vi "Signal_acquisition_v5.vi"() -> ()   [LabVIEW 2015]
uses:
  <vilib>/measure/madcrms.llb/Basic Averaged DC-RMS for 1 Chan.vi
  <vilib>/measure/matone.llb/Extract Single Tone Information 1 Chan.vi
  <vilib>/express/express arith-compare/Formula/XNode/ExpressFormulaBlockNode.xnode
  <vilib>/measure/NI_MAPro.lvlib
panel:
  in  "timeout ms":i32=2000
  in  "timeout ms\n (2000)":i32=2000
  in  "timeout ms\n (2000) 2":i32=2000
  in  "Delay\n (# Samples)":i32 max=16348
  in  "Trigger Level \n(0 mV)":i32
  out "DC value 2":dbl format="%0.2p"
  out "detected \nfrequency 2":dbl format="%.2p"
  out "Ieration\nnumber":i32
  out "millisecond \ntimer value":u32
  out "millisecond \nbegin timer":u32
  out "millisecond \nfinal timer":u32
  in  "Tab Control":T1(tab)
  out "Voltage Gain / Frequency":cluster{i32, dbl}[](graph)
  out "Cutoff Freqs (Hz)":i32[](array[numeric])
  in  "MEASURE AMPLITUD":bool
  out "Acquisition\ntime complete":u32
  out "MEASURED \namplitud":dbl format="%.2p"
  out "RESULT \nin amplittude":dbl
  out "FRECUENCY \nEND":i32
  out "detected \nphase (deg)":dbl format="%.2p"
  out "detected \nfrequency":dbl format="%.2p"
  in  "Filename":path=path "test.xlsx"
  in  "Trigger Mode":string(combo)="CH1_NE"
  in  "input":u16=1
  in  "Pause \nfor buffer (ms)":u32=100
  out "error out":errorcluster
  in  "VOLTS":dbl=0.1
  in  "FREQ END":i32=70000
  in  "FREQ START":i32=10000
  in  "number \nof intervals":i32=60
  in  "IP address":string="192.168.0.10"
  in  "Decimation":u16(ring)=8 items=["65536"=65535, "8192"=8192, "1024"=1024, "64"=64, "8"=8, "1"=1]
  in  "error in":errorcluster
  out "REAL TIME MEASUREMENT":dbl[](graph)
  in  "FREQ START 5":i32
  in  "number of intervals  3":i32
  in  "number of intervals  2":i32
  # "FREQUENCY SWEEP"
  # "FREQUENCY SWEEP"
  # "Settings parameters"
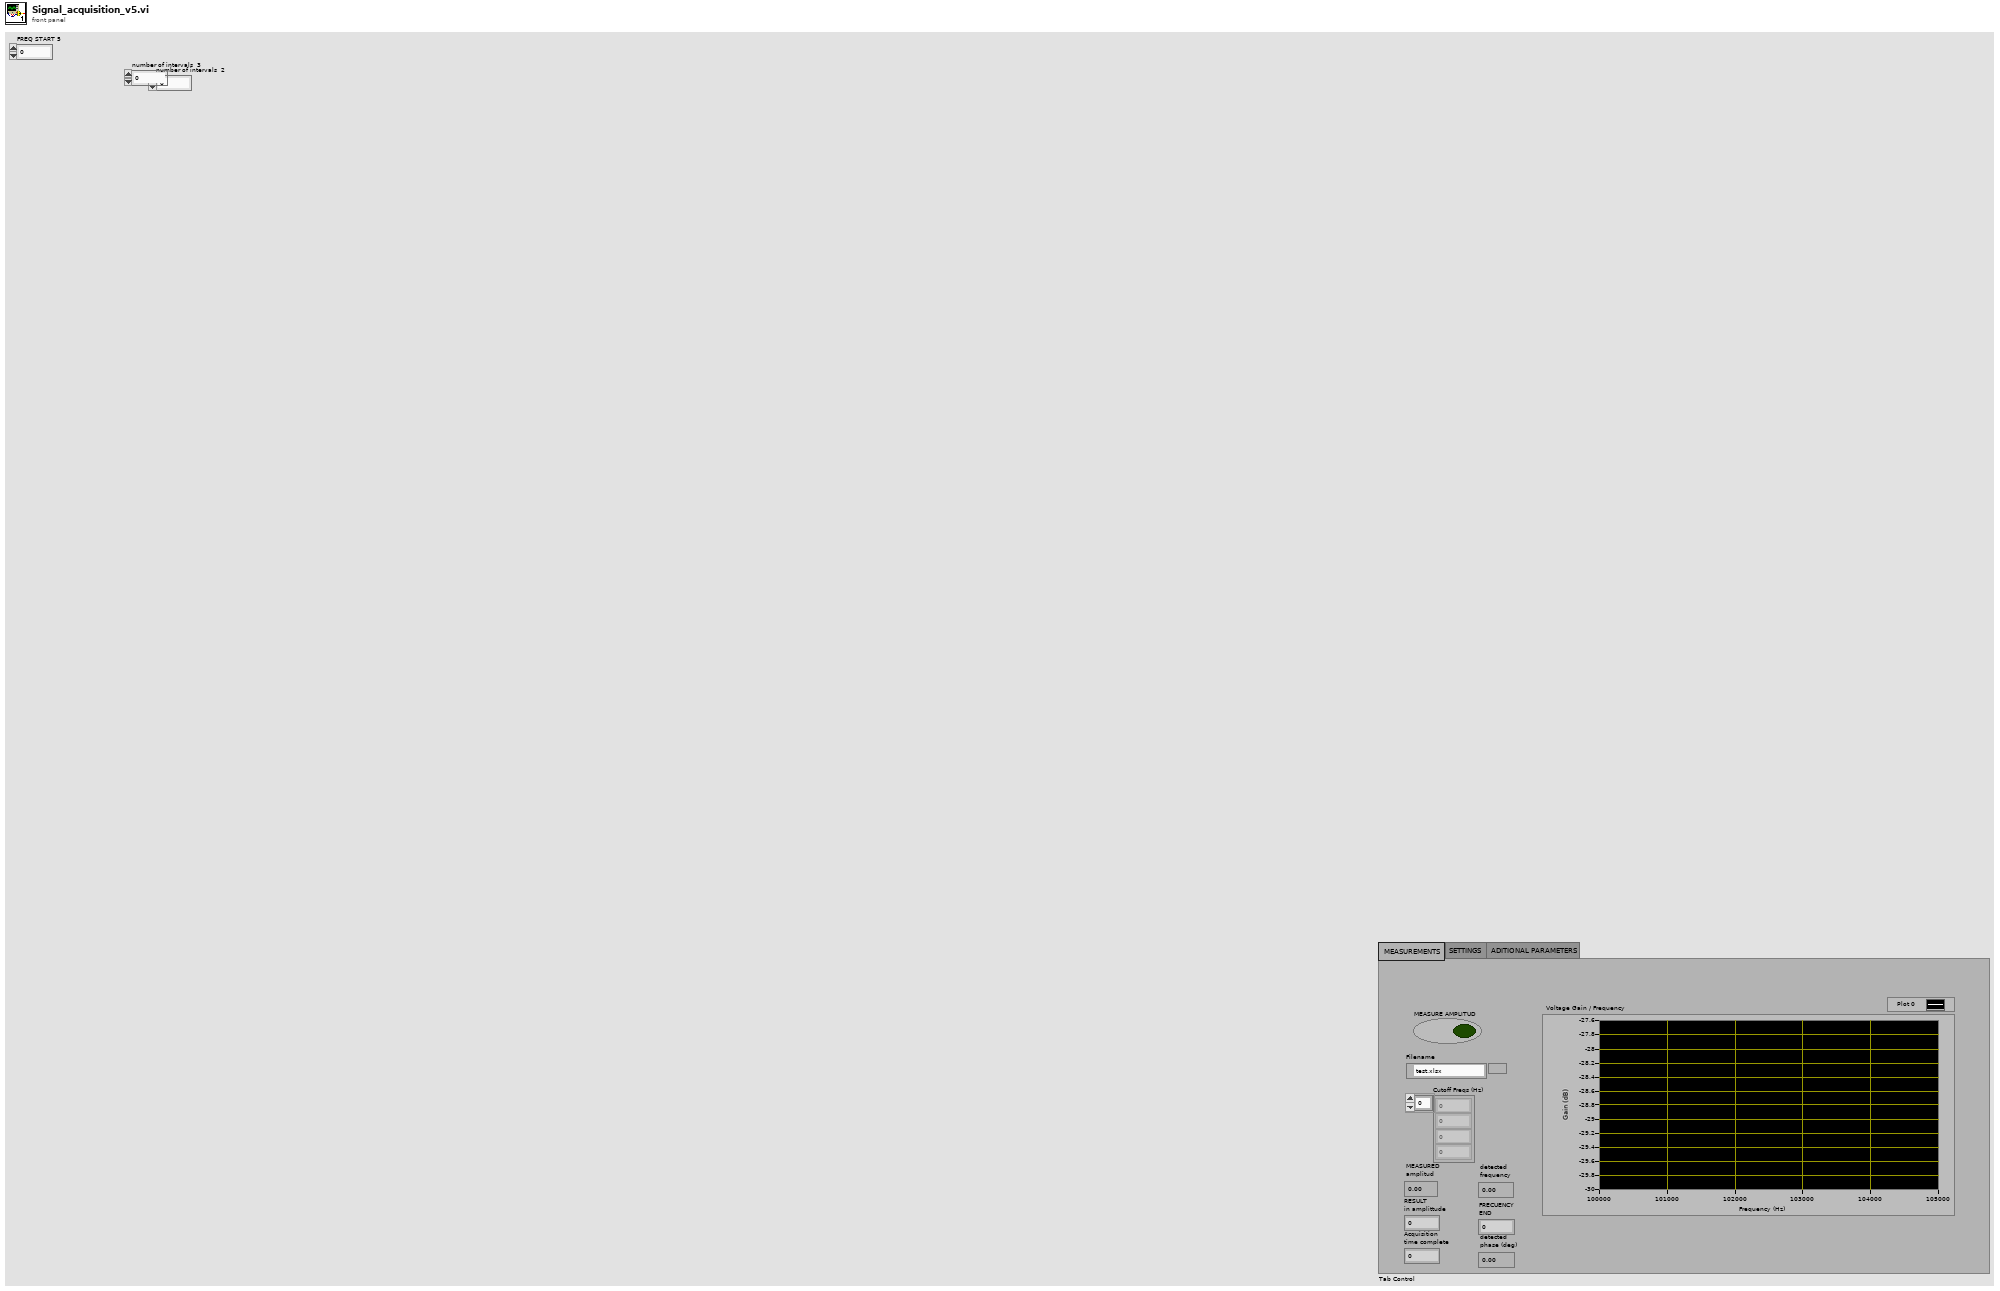
[diagram p1: front panel]
types:
  T1 = enum32{"MEASUREMENTS ", "SETTINGS", "ADITIONAL PARAMETERS"}
  T2 = enum16{"Standard", "Buffered", "CRLF", "Immediate"}
  T3 = enum32{"none", "input signal", "detected signal", "residual signal"}
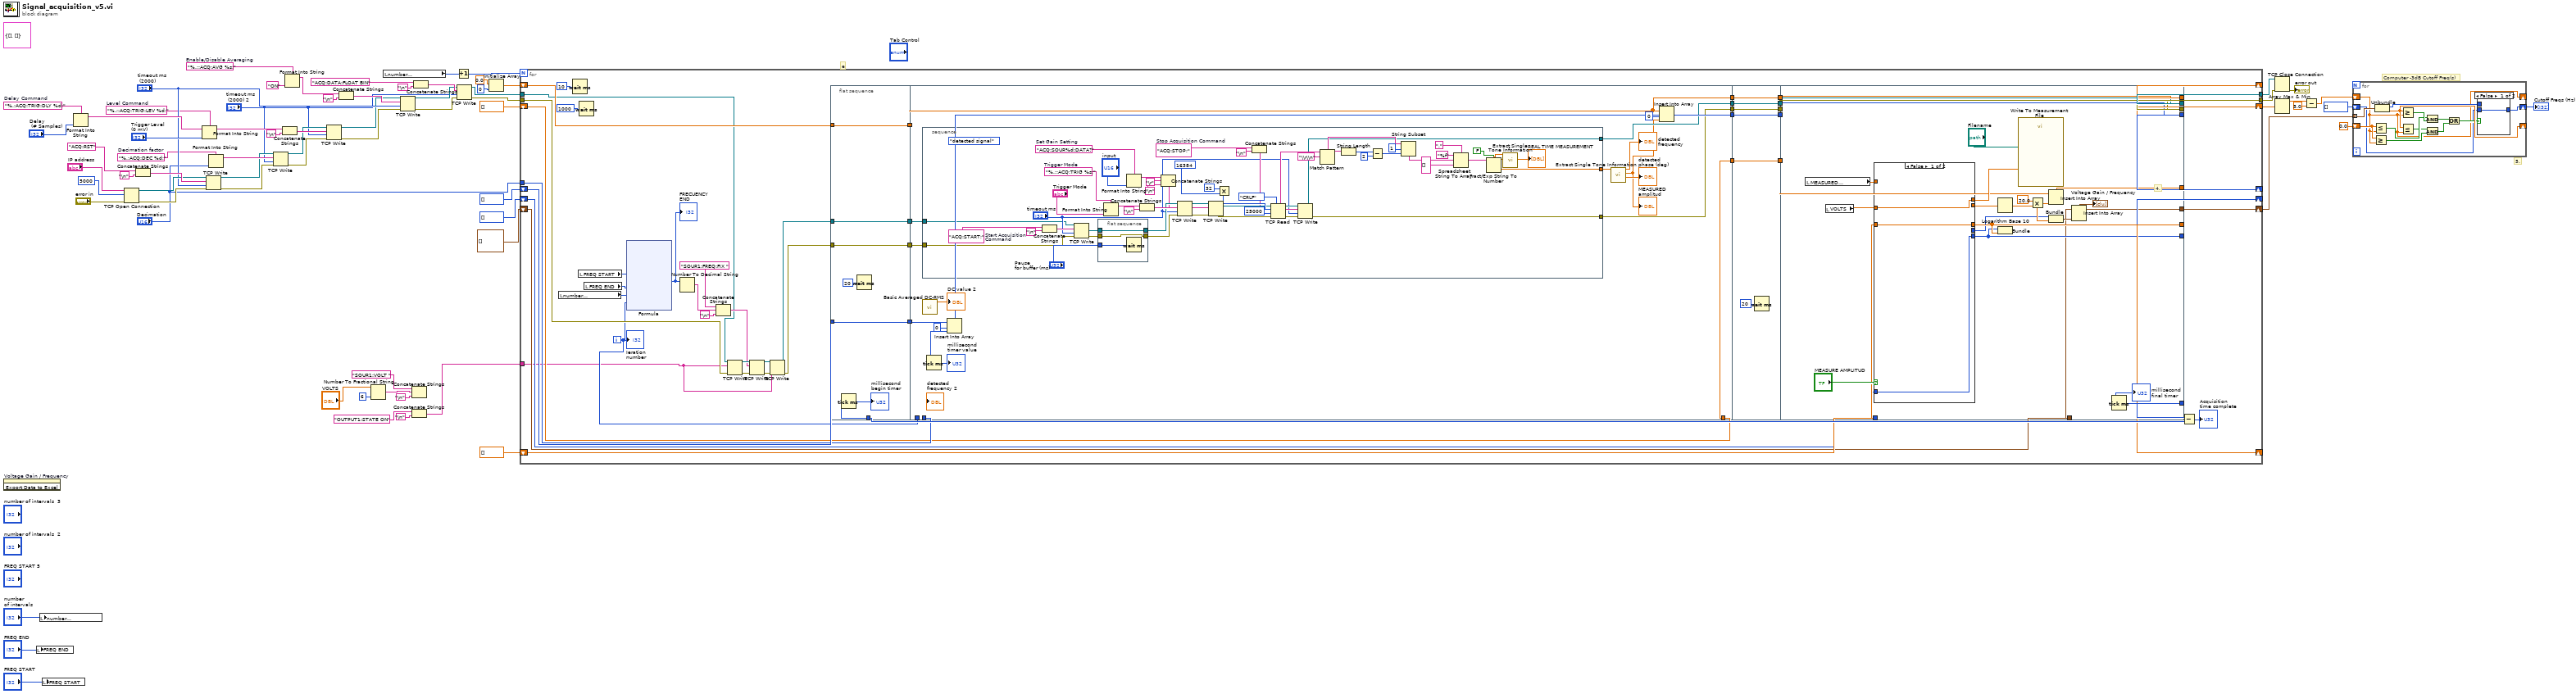
[diagram p0: block diagram]
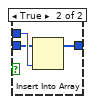
[diagram p2: hidden frame]
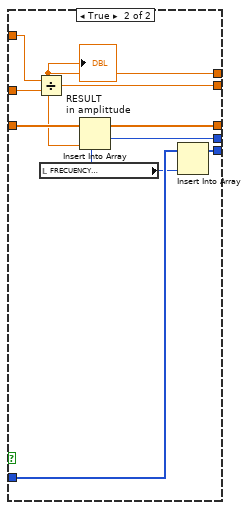
[diagram p3: hidden frame]
diagram:
  (unwired) cluster{dbl[], dbl[]} {[], []} ("FRECUENCY SWEEP")
  w37 = "%.;:ACQ:AVG %s;"  # Enable/Disable Averaging
  w45 = "%.;ACQ:DEC %d;"  # Decimation factor
  w46 = "%.;ACQ:TRIG:DLY %d;"  # Delay Command
  w47 = "%.;:ACQ:TRIG:LEV %d;"  # Level Command
  # "5."
  # "Computer -3dB Cutoff Freq(s)"
  # "e"
  n1 = invoke on="Voltage Gain / Frequency" class="XYGraph (strict)" method="Export Data to Excel"() -> ()  [unwired: 3 in, 3 out]
  n2 = local write "FREQ END"("FREQ END") -> ()
  n3 = local write "number \nof intervals"("number \nof intervals") -> ()
  n4 = local write "FREQ START"("FREQ START") -> ()
  n5 = Format Into String(format string=w46, "Delay\n (# Samples)") -> (resulting string=w65:string)  [unwired: 2 in, 1 out]
  n6 = TCP Open Connection(address="IP address", remote port or service name=u16 5000, error in (no error)="error in") -> (connection ID=w59:refnum<k5>, error out=w58:errorcluster)  [unwired: 2 in]
  n7 = Concatenate Strings("ACQ:RST" ("SCPI Message"), "\n") -> (w61:string)
  n8 = Format Into String(format string=w47, initial string=w65, "Trigger Level \n(0 mV)") -> (resulting string=w62:string)  [unwired: 1 in, 1 out]
  n9 = TCP Write(connection ID=w59, data in=w61, error in (no error)=w58, 9:"timeout ms\n (2000)") -> (connection ID out=w43:refnum<k5>, error out=w42:errorcluster)  [unwired: 1 out]
  n10 = Format Into String(format string=w45, "Decimation") -> (resulting string=w44:string)  [unwired: 2 in, 1 out]
  n11 = TCP Write(connection ID=w43, data in=w44, error in (no error)=w42, 9:"timeout ms\n (2000) 2") -> (connection ID out=w41:refnum<k5>, error out=w40:errorcluster)  [unwired: 1 out]
  n12 = Concatenate Strings(w62, "\n") -> (w56:string)
  n13 = Format Into String(format string=w37, "ON") -> (resulting string=w68:string)  [unwired: 2 in, 1 out]
  n14 = TCP Write(connection ID=w41, data in=w56, error in (no error)=w40, 9:"timeout ms\n (2000) 2") -> (connection ID out=w39:refnum<k5>, error out=w38:errorcluster)  [unwired: 1 out]
  n15 = Concatenate Strings(w68, "\n") -> (w57:string)
  n16 = Number To Fractional String(number="VOLTS", precision (6)=i16 6) -> (F-format string=w7:string)  [unwired: 2 in]
  n17 = local read "number \nof intervals"() -> (w23:i32)
  n18 = TCP Write(connection ID=w39, data in=w57, error in (no error)=w38, 9:"timeout ms\n (2000)") -> (connection ID out=w35:refnum<k5>, error out=w34:errorcluster)  [unwired: 1 out]
  n19 = Concatenate Strings("SOUR1:VOLT " ("SCPI Message"), w7, "\n") -> ()  [unwired: 1 out]
  n20 = Concatenate Strings("OUTPUT1:STATE ON" ("SCPI Message"), "\n") -> (w1:string)
  n21 = Concatenate Strings("ACQ:DATA:FLOAT BIN" ("SCPI Message"), "\n") -> (w53:string)
  n22 = Increment(x=w23) -> (x+1=w22:i32)
  n23 = TCP Write(connection ID=w35, data in=w53, error in (no error)=w34, 9:"timeout ms\n (2000) 2") -> (connection ID out=w32:refnum<k5>, error out=w31:errorcluster)  [unwired: 1 out]
  n24 = Initialize Array(0.0 ("element"), 0 ("dimension size")) -> (w26:dbl[])
  n25 = for {
    N: w22 -> [_]
    tunnel: w32 -> [w103]
    tunnel: [w121] -> w52
    tunnel: [w120] -> w51
    tunnel: w31 -> [w100]
    shift-right: [w123] -> _
    shift-left: u32[] [] -> [w122]
    tunnel: "Decimation" -> [w113]
    shift-right: [w111] -> _
    shift-left: w26 -> [w109]
    shift-right: [w96] -> _
    shift-left: dbl[] [] -> [w97]
    shift-right: [w92] -> _
    shift-left: i32[] [] -> [w91]
    shift-right: [w87] -> w11
    shift-left: dbl[] [] -> [w86]
    shift-right: [w85] -> w10
    shift-left: cluster{"FRECUENCY END":i32, dbl}[] [] -> [w84]
    tunnel: w1 -> [w72]
    i -> [w73]
    n26 = local read "number \nof intervals"() -> (w93:i32)
    n27 = Wait (ms)(milliseconds to wait=u32 10) -> ()  [unwired: 1 out]
    n28 = local read "FREQ START"() -> (w94:i32)
    n29 = Wait (ms)(milliseconds to wait=u32 1000) -> ()  [unwired: 1 out]
    n30 = local read "FREQ END"() -> (w95:i32)
    n31 = xnode "Formula"("Fin"=w94, "Fend"=w95, "Ninter"=w93, "i"=w73) -> ("Result"=w88:i32)  [unwired: 1 in, 1 out]
    "FRECUENCY \nEND" <- w88
    n32 = Number To Decimal String(number=w88) -> (decimal integer string=w98:string)  [unwired: 1 in]
    n33 = Concatenate Strings("SOUR1:FREQ:FIX " ("SCPI Message"), w98, "\n") -> (w104:string)
    n34 = TCP Write(connection ID=w103, data in=w72, error in (no error)=w100) -> (connection ID out=w107:refnum<k5>, error out=w106:errorcluster)  [unwired: 1 in, 1 out]
    n35 = TCP Write(connection ID=w107, data in=w104, error in (no error)=w106) -> (connection ID out=w90:refnum<k5>, error out=w89:errorcluster)  [unwired: 1 in, 1 out]
    n36 = TCP Write(connection ID=w90, data in=w72, error in (no error)=w89) -> (connection ID out=w102:refnum<k5>, error out=w101:errorcluster)  [unwired: 1 in, 1 out]
    n37 = flat-sequence {
      tunnel: w122 -> [w141]
      tunnel: w101 -> [w142]
      tunnel: w102 -> [w143]
      tunnel: [w143] -> w119
      tunnel: [w142] -> w118
      tunnel: [w141] -> w117
      tunnel: [w140] -> w115
      tunnel: [w139] -> w110
      tunnel: w109 -> [w139]
      tunnel: [w155] -> w83
      tunnel: [w153] -> w81
      tunnel: [w152] -> w79
      tunnel: w119 -> [w159]
      tunnel: w118 -> [w158]
      tunnel: w117 -> [w154]
      tunnel: w113 -> [_]
      tunnel: [w148] -> w77
      tunnel: w73 -> [_]
      tunnel: w110 -> [w148]
      tunnel: w86 -> [w144]
      tunnel: [w144] -> w75
      tunnel: w83 -> [w220]
      tunnel: [w220] -> w82
      tunnel: w81 -> [w219]
      tunnel: [w219] -> w80
      tunnel: w79 -> [w218]
      tunnel: [w218] -> w78
      tunnel: w77 -> [w217]
      tunnel: [w217] -> w76
      tunnel: w75 -> [w216]
      tunnel: [w216] -> w74
      tunnel: [w242] -> w120
      tunnel: [w243] -> w121
      tunnel: [w244] -> w123
      tunnel: w82 -> [w244]
      tunnel: w80 -> [w243]
      tunnel: w78 -> [w242]
      tunnel: [w241] -> w116
      tunnel: w76 -> [w240]
      tunnel: [w240] -> w111
      tunnel: w97 -> [w236]
      tunnel: [w234] -> w96
      tunnel: [w233] -> w92
      tunnel: w91 -> [w235]
      tunnel: [w228] -> w87
      tunnel: w74 -> [w227]
      tunnel: [w225] -> w85
      tunnel: w84 -> [w224]
      frame #0 {
        n38 = Tick Count (ms)() -> (millisecond timer value=w140:u32)
        "millisecond \nbegin timer" <- w140
        n39 = Wait (ms)(milliseconds to wait=u32 20) -> ()  [unwired: 1 out]
      }
      frame #1 {
        n40 = stacked-sequence {
          tunnel: w159 -> [w161]
          tunnel: w158 -> [w164]
          tunnel: [w162] -> w153
          tunnel: [w163] -> w152
          tunnel: [w160] -> w146
          frame #0 {
            w171 = "ACQ:STOP;"  # Stop Acquisition Command
            (unwired) T3."detected signal" ("export mode")
            w181 = "ACQ:SOUR%d:DATA?"  # Set Gain Setting
            w208 = "%.;:ACQ:TRIG %s;"  # Trigger Mode
            w210 = "ACQ:START;"  # Start Acquisition Command
            n41 = Concatenate Strings(w210, "\n") -> (w211:string)
            n42 = TCP Write(connection ID=w161, data in=w211, error in (no error)=w164, 9:"timeout ms") -> (connection ID out=w185:refnum<k5>, error out=w184:errorcluster)  [unwired: 1 out]
            n43 = flat-sequence {
              tunnel: "Pause \nfor buffer (ms)" -> [w214]
              tunnel: [w213] -> w183
              tunnel: [w212] -> w182
              tunnel: w185 -> [w213]
              tunnel: w184 -> [w212]
              frame #0 {
                n44 = Wait (ms)(milliseconds to wait=w214) -> ()  [unwired: 1 out]
              }
            }
            n45 = Format Into String(format string=w208, "Trigger Mode") -> (resulting string=w205:string)  [unwired: 2 in, 1 out]
            n46 = Format Into String(format string=w181, "input") -> (resulting string=w179:string)  [unwired: 2 in, 1 out]
            n47 = Concatenate Strings(w205, "\n") -> (w206:string)
            n48 = Concatenate Strings(w179, "\r", "\n") -> (w178:string)
            n49 = TCP Write(connection ID=w183, data in=w206, error in (no error)=w182, 9:"timeout ms") -> (connection ID out=w176:refnum<k5>, error out=w175:errorcluster)  [unwired: 1 out]
            n50 = TCP Write(connection ID=w176, data in=w178, error in (no error)=w175) -> (connection ID out=w177:refnum<k5>, error out=w174:errorcluster)  [unwired: 1 in, 1 out]
            n51 = Multiply(x=32, y=16384 ("bytes to read")) -> (x*y=w186:i32)
            n52 = Concatenate Strings(w171, "\n") -> (w169:string)
            n53 = TCP Read(connection ID=w177, bytes to read=w186, error in (no error)=w174, 7:T2."CRLF" ("mode (standard)"), 9:25000 ("timeout ms (25000)")) -> (connection ID out=w172:refnum<k5>, data out=w187:string, error out=w168:errorcluster)
            n54 = TCP Write(connection ID=w172, data in=w169, error in (no error)=w168, 9:"timeout ms") -> (connection ID out=w162:refnum<k5>, error out=w163:errorcluster)  [unwired: 1 out]
            n55 = Match Pattern(string=w187, regular expression="\\r\\n") -> (before substring=w193:string)  [unwired: 1 in, 3 out]
            n56 = String Length(string=w193) -> (length=w196:i32)
            n57 = Subtract(x=w196, y=2) -> (x-y=w197:i32)
            n58 = String Subset(string=w193, offset (0)=1, length (rest)=w197) -> (substring=w194:string)
            n59 = Spreadsheet String To Array(delimiter (Tab)=",", format string="%f", spreadsheet string=w194, array type (2D Dbl)=string[] [] ("Array")) -> (array=w200:string[])
            n60 = Fract/Exp String To Number(use system decimal point (T)=FALSE, string=w200) -> (number=w160:dbl[])  [unwired: 3 out]
            "REAL TIME MEASUREMENT" <- w160
            n61 = call-poly <vilib>:"Extract Single Tone Information.vi"("time signal in"=w160) -> ()  [unwired: 5 in, 6 out]
          }
        }
        n62 = call-poly <vilib>:"Basic Averaged DC-RMS.vi"() -> ("DC value"=→"DC value 2":dbl)  [unwired: 8 in, 3 out]
        n63 = Tick Count (ms)() -> (millisecond timer value=w156:u32)
        "millisecond \ntimer value" <- w156
        n64 = Insert Into Array(array=w154, index=0, new element=w156) -> (w155:u32[])
        n65 = call-poly <vilib>:"Extract Single Tone Information.vi"("time signal in"=w146) -> ("detected phase (deg)"=→"detected \nphase (deg)":dbl, "detected amplitude"=w145:dbl, "detected frequency"=→"detected \nfrequency":dbl)  [unwired: 5 in, 3 out]
        "MEASURED \namplitud" <- w145
        n66 = Insert Into Array(array=w148, index=0, new element=w145) -> ()  [unwired: 1 out]
      }
      frame #2 {
        n67 = Wait (ms)(milliseconds to wait=u32 20) -> ()  [unwired: 1 out]
      }
      frame #3 {
        # "4."
        n68 = local read "MEASURED \namplitud"() -> (w239:dbl)
        n69 = local read "VOLTS"() -> (w222:dbl)
        n70 = case shown="False" "MEASURE AMPLITUD" {
          tunnel: w239 -> [_ w251]
          tunnel: [w245 w250] -> w237
          tunnel: w236 -> [w247 w255]
          tunnel: [w247 w254] -> w234
          tunnel: [w246 w253] -> w233
          tunnel: w235 -> [w246 w252]
          tunnel: [_ w250] -> w223
          tunnel: [_ w249] -> w226
          tunnel: w222 -> [w245 w248]
          frame False {
          }
          frame True {
            n71 = Divide(x=w251, y=w248) -> (x/y=w250:dbl)
            "RESULT \nin amplittude" <- w250
            n72 = local read "FRECUENCY \nEND"() -> (w249:i32)
            n73 = Insert Into Array(array=w255, new element=w250) -> (w254:dbl[])  [unwired: 1 in]
            n74 = Insert Into Array(array=w252, new element=w249) -> (w253:i32[])  [unwired: 1 in]
          }
        }
        n75 = Logarithm Base 10(1:w223) -> (0:w230:dbl)
        n76 = Bundle(w233, w234) -> ()  [unwired: 1 in, 1 out]
        n77 = call "Write To Measurement File"("Signals"=w237, "Filename"="Filename") -> ()  [unwired: 15 in, 3 out]
        n78 = Multiply(x=20.0, y=w230) -> (x*y=w229:dbl)
        n79 = Insert Into Array(array=w227, new element=w229) -> (w228:dbl[])  [unwired: 1 in]
        n80 = Bundle("FRECUENCY \nEND"=w226, w229) -> (w232:cluster{"FRECUENCY \nEND":i32, dbl})  [unwired: 1 in]
        n81 = Insert Into Array(array=w224, new element=w232) -> (w225:cluster{"FRECUENCY END":i32, dbl}[])  [unwired: 1 in]
        "Voltage Gain / Frequency" <- w225
        n82 = Tick Count (ms)() -> (millisecond timer value=w241:u32)
        "millisecond \nfinal timer" <- w241
      }
    }
    n83 = Subtract(x=w116, y=w115) -> (x-y=→"Acquisition\ntime complete":u32)
    "Ieration\nnumber" <- w73
  }
  n84 = TCP Close Connection(connection ID=w52, error in (no error)=w51) -> (error out=→"error out":errorcluster)  [unwired: 1 in, 1 out]
  n85 = Array Max & Min(array=w11) -> (max value=w12:dbl)  [unwired: 3 out]
  n86 = Subtract(x=w12, y=3.0) -> (x-y=w13:dbl)
  n87 = for {
    tunnel: w10 -> [w269] mode=indexing
    shift-right: [w263] -> _
    shift-left: 0.0 -> [w264]
    shift-right: [w257] -> w15
    shift-left: i32[] [] -> [w258]
    shift-right: [w256] -> _
    shift-left: w13 -> [w256]
    n88 = Less Or Equal?(x=w264, y=w256) -> (x <= y?=w267:bool)
    n89 = Greater Or Equal?(x=w264, y=w256) -> (x >= y?=w265:bool)
    n90 = Unbundle(w269) -> ("FRECUENCY END"=w259:i32, w263:dbl)
    n91 = Greater Or Equal?(x=w263, y=w256) -> (x >= y?=w268:bool)
    n92 = Less Or Equal?(x=w263, y=w256) -> (x <= y?=w266:bool)
    n93 = And(x=w267, y=w268) -> (x .and. y?=w261:bool)
    n94 = And(x=w266, y=w265) -> (x .and. y?=w262:bool)
    n95 = Or(x=w261, y=w262) -> (x .or. y?=w260:bool)
    n96 = case shown="False" w260 {
      tunnel: w259 -> [_ w273]
      tunnel: w258 -> [w270 w272]
      tunnel: [w270 w271] -> w257
      frame False {
      }
      frame True {
        n97 = Insert Into Array(array=w272, new element=w273) -> (w271:i32[])  [unwired: 1 in]
      }
    }
  }
  "Cutoff Freqs (Hz)" <- w15
